vi "acq_loop.vi"(8 "Marker Queue":refnum<queue>, 9 "Log queue":refnum<queue>, 10 "Server queue":refnum<queue>, 11 "Message Queues":T2) -> (0 "error out":errorcluster)   [LabVIEW 2013]
doc: "Message loop for handling messages pertaining to the acquisition of data from the hardware."
uses:
  queues/que_all_message_queues.ctl
  queues/que_message_cluster.ctl
  gui/type_def/device.ctl
  acq_state.ctl
  queues/que_enqueue_message_single.vi
  <vilib>/Utility/error.llb/Error Cluster From Error Code.vi
  <vilib>/ErrorRing/Error Ring.xnode
panel:
  out "eeg_device":T1
  in  "error in (no error)":errorcluster
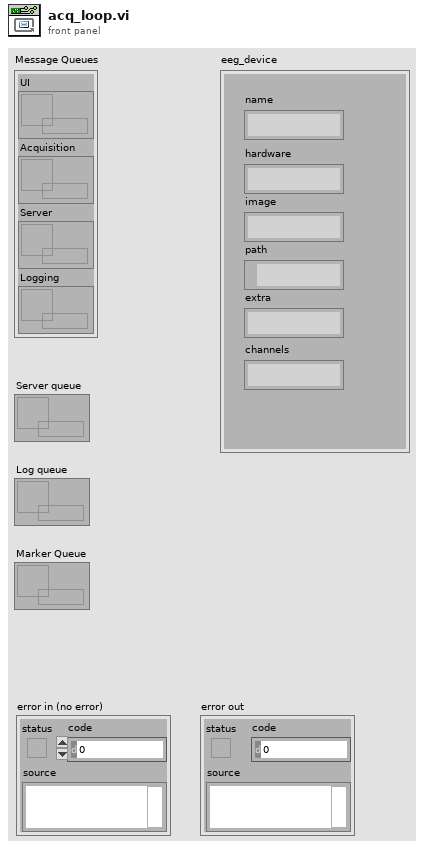
[diagram p1: front panel]
types:
  T1 = typedef "device.ctl" = cluster{"name":string, "hardware":string, "image":string, "path":path, "extra":string, "channels":string}
  T2 = typedef "que_all_message_queues.ctl" = cluster{"UI":refnum<queue>, "Acquisition":refnum<queue>, "Server":refnum<queue>, "Logging":refnum<queue>}
  T3 = typedef "acq_state.ctl" = enum16{"Idle", "Acquiring"}
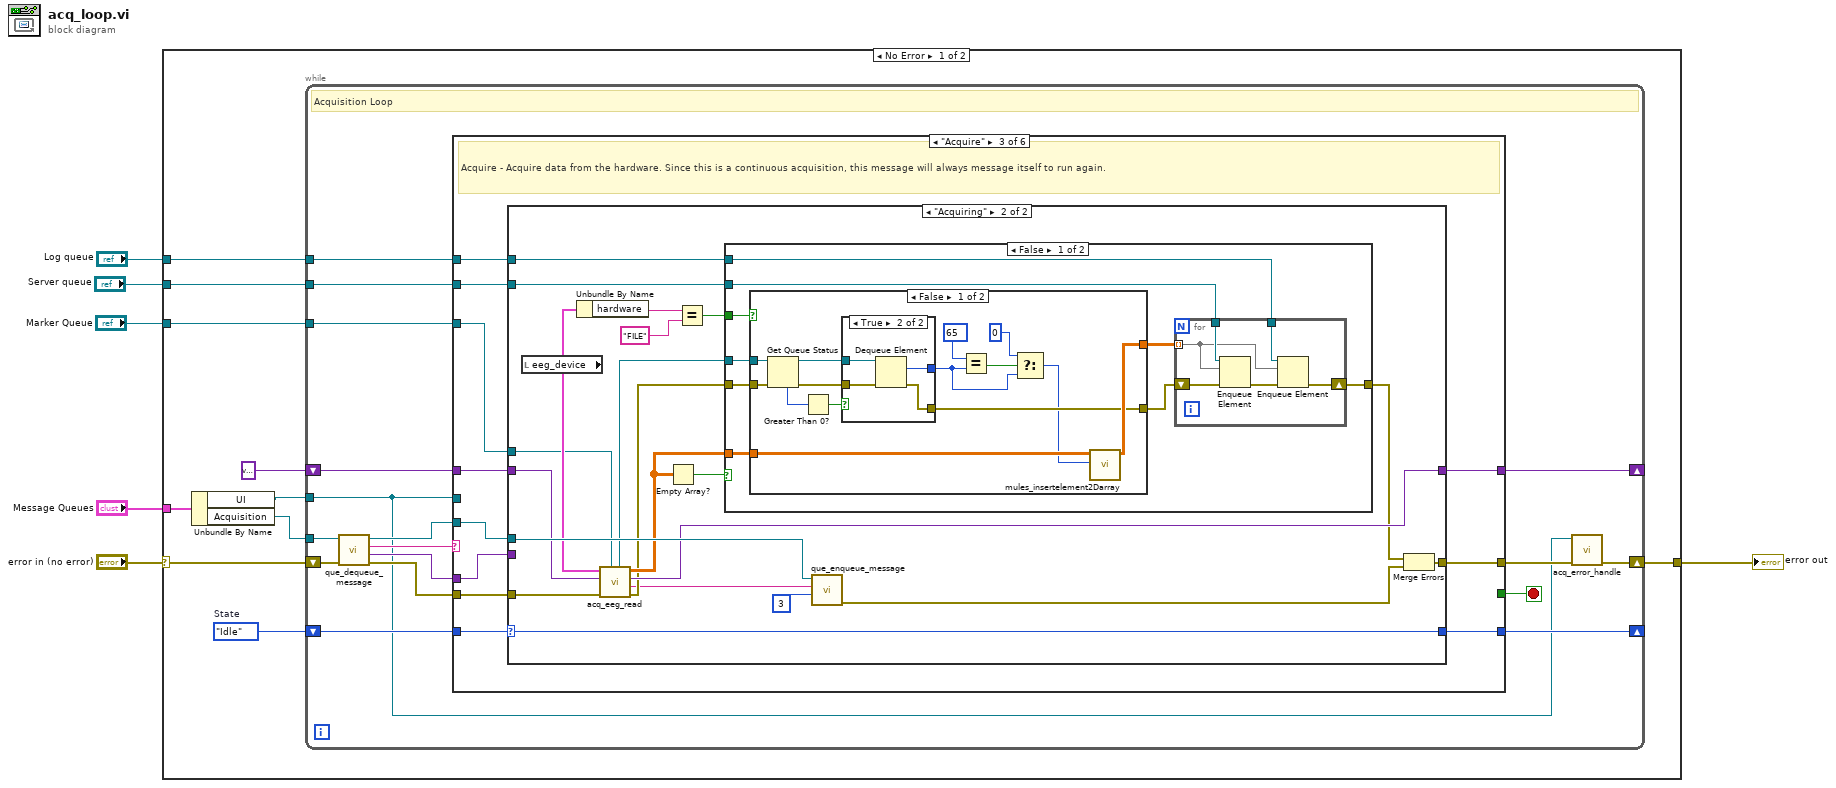
[diagram p0: block diagram]
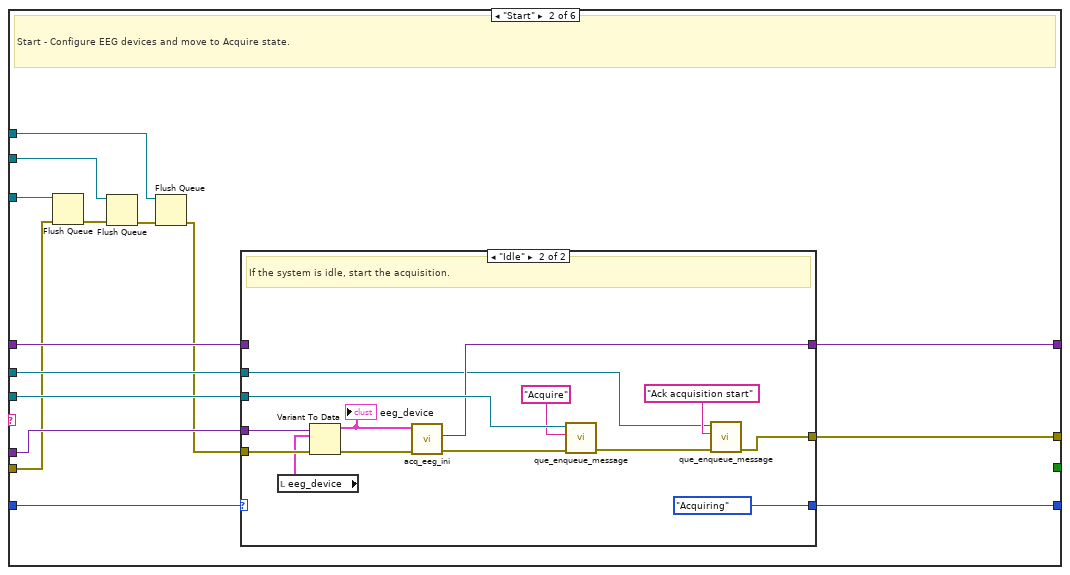
[diagram p3: hidden frame]
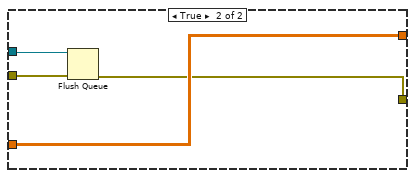
[diagram p7: hidden frame]
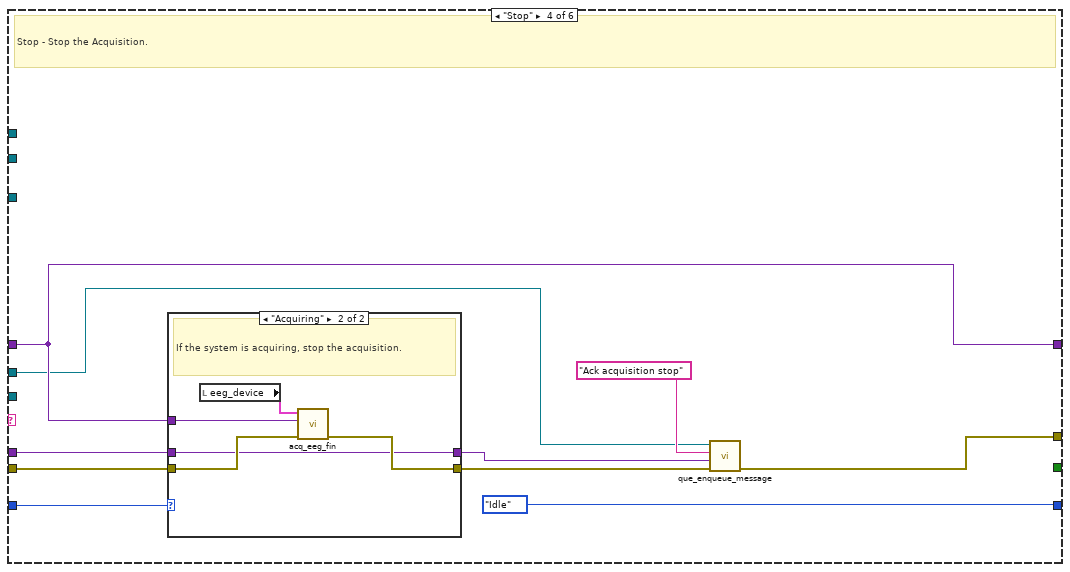
[diagram p9: hidden frame]
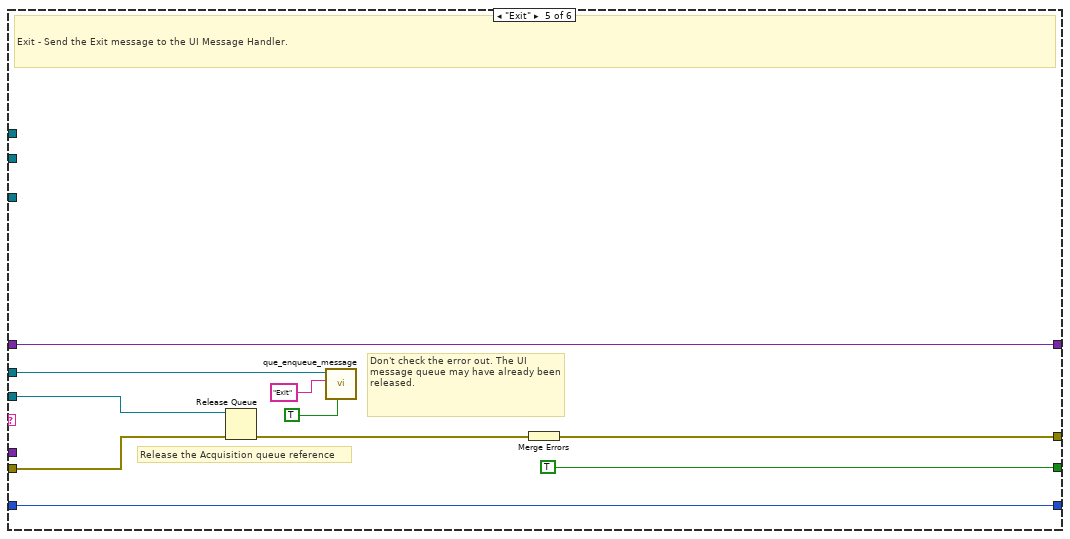
[diagram p11: hidden frame]
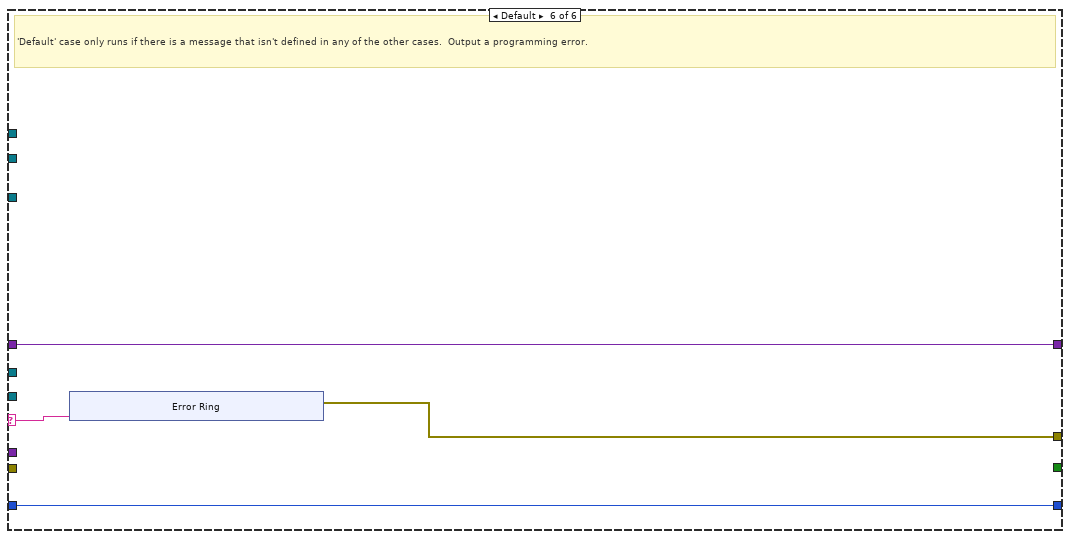
[diagram p12: hidden frame]
diagram:
  n1 = case shown="No Error" "error in (no error)" {
    selector: "error in (no error)" -> [w13 w180]
    tunnel: "Message Queues" -> [w16 _]
    tunnel: [w14 w180] -> w5
    tunnel: "Marker Queue" -> [w9 _]
    tunnel: "Server queue" -> [w8 _]
    tunnel: "Log queue" -> [w7 _]
    frame No Error {
      w11 = acq_state."Idle"  # State
      n2 = Unbundle By Name(w16) -> ("UI"=w12:refnum<queue>, "Acquisition"=w15:refnum<queue>)
      n3 = while {
        tunnel: w15 -> [w28]
        shift-right: [w25] -> w14
        shift-left: w13 -> [w32]
        tunnel: w12 -> [w22]
        shift-right: [w26] -> _
        shift-left: w11 -> [w27]
        shift-right: [w17] -> _
        shift-left: variant ("Variant out") -> [w21]
        tunnel: w9 -> [w20]
        tunnel: w8 -> [w19]
        tunnel: w7 -> [w18]
        stop <- w33 stop-if-true
        # "Acquisition Loop"
        n4 = call "que_dequeue_message.vi"("error in (no error)"=w32, "Message Queue"=w28) -> ("error out"=w31:errorcluster, "Message Data"=w29:variant, "Message"=w30:string, "dup Message Queue"=w23:refnum<queue>)  [unwired: 6 in]
        n5 = case "Message Cases" shown="\"Acquire\"" w30 {
          selector: w30 -> [_ _ _ _ _ w170]
          tunnel: w23 -> [_ w50 w78 _ w161 _]
          tunnel: w31 -> [w34 w39 w77 w151 w165 _]
          tunnel: [w34 w51 w79 w145 w167 w171] -> w24
          tunnel: [_ _ _ _ TRUE _] -> w33
          tunnel: w29 -> [_ w47 w74 w143 _ _]
          tunnel: w22 -> [_ w45 _ w146 w166 _]
          tunnel: w27 -> [w36 w48 w75 w150 w160 w172]
          tunnel: [w36 w49 w76 acq_state."Idle" ("State") w160 w172] -> w26
          tunnel: [w35 w46 w73 w149 w159 w169] -> w17
          tunnel: w21 -> [w35 w44 w72 w149 w159 w169]
          tunnel: w20 -> [_ w42 w71 _ _ _]
          tunnel: w19 -> [_ w43 w70 _ _ _]
          tunnel: w18 -> [_ w41 w69 _ _ _]
          frame "Initialize" {
            # "Initialize  - Initialize is currently a no-op.  The EEG initialization is done with the 'start' message."
          }
          frame "Start" {
            # "Start - Configure EEG devices and move to Acquire state."
            n6 = Flush Queue(queue=w42, error in (no error)=w39) -> (error out=w40:errorcluster)  [unwired: 2 out]
            n7 = Flush Queue(queue=w43, error in (no error)=w40) -> (error out=w38:errorcluster)  [unwired: 2 out]
            n8 = Flush Queue(queue=w41, error in (no error)=w38) -> (error out=w37:errorcluster)  [unwired: 2 out]
            n9 = case shown="\"Idle\"" w48 {
              selector: w48 -> [w53 _]
              tunnel: [w54 w59] -> w51
              tunnel: w37 -> [w54 w64]
              tunnel: w50 -> [_ w68]
              tunnel: [w53 acq_state."Acquiring" ("Acquisition State")] -> w49
              tunnel: w47 -> [_ w65]
              tunnel: [w52 w61] -> w46
              tunnel: w45 -> [_ w58]
              tunnel: w44 -> [w52 _]
              frame "Acquiring" {
                # "The system is already acquiring. Ignore the \"Start\" message."
              }
              frame "Idle" {
                # "If the system is idle, start the acquisition."
                n10 = local read "eeg_device"() -> (w63:T1)
                n11 = Variant To Data(error in=w64, type=w63, Variant=w65) -> (data=w57:T1, error out=w62:errorcluster)
                "eeg_device" <- w57
                n12 = call "acq_eeg_ini.vi"("error in (no error)"=w62, "eeg_device in"=w57) -> ("error out"=w55:errorcluster, "Variant"=w61:variant)  [unwired: 8 in]
                n13 = call-poly "que_enqueue_message.vi"("error in (no error)"=w55, "Message"="Acquire", "Message Queue"=w68) -> ("error out"=w56:errorcluster)  [unwired: 7 in, 1 out]
                n14 = call-poly "que_enqueue_message.vi"("error in (no error)"=w56, "Message"="Ack acquisition start", "Message Queue"=w58) -> ("error out"=w59:errorcluster)  [unwired: 7 in, 1 out]
              }
            }
          }
          frame "Acquire" {
            # "Acquire - Acquire data from the hardware. Since this is a continuous acquisition, this message will always message itself to run again."
            n15 = case shown="\"Acquiring\"" w75 {
              selector: w75 -> [w81 w89]
              tunnel: [w82 w102] -> w79
              tunnel: w78 -> [_ w101]
              tunnel: w77 -> [w82 w96]
              tunnel: [w81 w89] -> w76
              tunnel: w74 -> [_ _]
              tunnel: [w80 w100] -> w73
              tunnel: w72 -> [w80 w99]
              tunnel: w71 -> [_ w88]
              tunnel: w70 -> [_ w95]
              tunnel: w69 -> [_ w85]
              frame "Idle", Default {
                # "Ignore \"Acquire\" messages when the acquisition is idle."
              }
              frame "Acquiring" {
                # "Acquire more data while in the \"Acquiring\" state."
                n16 = local read "eeg_device"() -> (w93:T1)
                n17 = Unbundle By Name(w93) -> ("hardware"=w92:string)
                n18 = call "acq_eeg_read.vi"("Marker Queue"=w88, "error in (no error)"=w96, "variant in"=w99, "eeg_device"=w93) -> ("Next Acq State"=w86:string, "Variant out"=w100:variant, "eeg samples"=w97:dbl[][], "Marker Queue Out"=w87:refnum<queue>)  [unwired: 3 in, 1 out]
                n19 = Empty Array?(array=w97) -> (empty?=w98:bool)
                n20 = Equal?(x=w92, y="FILE" ("Message")) -> (x = y?=w90:bool)
                n21 = case shown="False" w98 {
                  tunnel: w97 -> [w111 _]
                  tunnel: w96 -> [w110 w141]
                  tunnel: w95 -> [w109 _]
                  tunnel: [w107 w141] -> w94
                  tunnel: w90 -> [w106 _]
                  tunnel: w87 -> [w104 _]
                  tunnel: w85 -> [w103 _]
                  frame False {
                    n22 = case shown="False" w106 {
                      tunnel: w111 -> [w131 w140]
                      tunnel: w110 -> [w126 w139]
                      tunnel: [w125 w140] -> w105
                      tunnel: [w124 w138] -> w108
                      tunnel: w104 -> [w123 w137]
                      frame False {
                        n23 = Get Queue Status(queue=w123, error in (no error)=w126) -> (queue out=w128:refnum<queue>, error out=w127:errorcluster, # elements in queue=w130:i32)  [unwired: 1 in, 5 out]
                        n24 = Greater Than 0?(x=w130) -> (x > 0?=w129:bool)
                        n25 = case shown="True" w129 {
                          tunnel: [w132 w136] -> w124
                          tunnel: w128 -> [_ w135]
                          tunnel: [_ w134] -> w120
                          tunnel: w127 -> [w132 w133]
                          frame False {
                          }
                          frame True {
                            n26 = Dequeue Element(queue=w135, error in (no error)=w133) -> (element=w134:u8, error out=w136:errorcluster)  [unwired: 1 in, 2 out]
                          }
                        }
                        n27 = Equal?(x=u8 65 ("y"), y=w120) -> (x = y?=w121:bool)
                        n28 = Select(t=u8 0, s=w121, f=w120) -> (s? t:f=w118:u8)
                        n29 = call "mules_insertelement2Darray.vi"("new element"=w118, "2D array in"=w131) -> ("2D array out"=w125:dbl[][])  [unwired: 9 in]
                      }
                      frame True {
                        n30 = Flush Queue(queue=w137, error in (no error)=w139) -> (error out=w138:errorcluster)  [unwired: 2 out]
                      }
                    }
                    n31 = for {
                      tunnel: w109 -> [w117]
                      tunnel: w105 -> [w113] mode=indexing
                      shift-right: [w112] -> w107
                      shift-left: w108 -> [w116]
                      tunnel: w103 -> [w114]
                      n32 = Enqueue Element(queue=w117, element=w113, error in (no error)=w116) -> (error out=w115:errorcluster)  [unwired: 1 in, 2 out]
                      n33 = Enqueue Element(queue=w114, element=w113, error in (no error)=w115) -> (error out=w112:errorcluster)  [unwired: 1 in, 2 out]
                    }
                  }
                  frame True {
                  }
                }
                n34 = call-poly "que_enqueue_message.vi"("Message Data"=3 ("t"), "Message"=w86, "Message Queue"=w101) -> ("error out"=w83:errorcluster)  [unwired: 7 in, 1 out]
                n35 = Merge Errors(w94, w83) -> (w102:errorcluster)
              }
            }
          }
          frame "Stop" {
            # "Stop - Stop the Acquisition."
            n36 = case shown="\"Acquiring\"" w150 {
              tunnel: w151 -> [w153 w158]
              tunnel: w149 -> [_ w157]
              tunnel: [w153 w155] -> w147
              tunnel: [w152 w154] -> w144
              tunnel: w143 -> [w152 w154]
              frame "Idle", Default {
                # "The system is already idle. Ignore the \"Stop\" message."
              }
              frame "Acquiring" {
                # "If the system is acquiring, stop the acquisition."
                n37 = local read "eeg_device"() -> (w156:T1)
                n38 = call "acq_eeg_fin.vi"("error in (no error)"=w158, "variant in"=w157, "eeg_device"=w156) -> ("error out"=w155:errorcluster)  [unwired: 8 in]
              }
            }
            n39 = call-poly "que_enqueue_message.vi"("error in (no error)"=w147, "Message Data"=w144, "Message"="Ack acquisition stop", "Message Queue"=w146) -> ("error out"=w145:errorcluster)  [unwired: 6 in, 1 out]
          }
          frame "Exit" {
            # "Don't check the error out. The UI message queue may have already been released."
            # "Release the Acquisition queue reference"
            # "Exit - Send the Exit message to the UI Message Handler."
            n40 = Release Queue(queue=w161, error in (no error)=w165) -> (error out=w162:errorcluster)  [unwired: 1 in, 2 out]
            n41 = call-poly "que_enqueue_message.vi"("Priority Message? (F)"=TRUE, "Message"="Exit", "Message Queue"=w166) -> ()  [unwired: 7 in, 2 out]
            n42 = Merge Errors(w162) -> (w167:errorcluster)
          }
          frame Default {
            # "'Default' case only runs if there is a message that isn't defined in any of the other cases.  Output a programming error."
            n43 = xnode "Error Ring"("parameter 0"=w170) -> ("error out"=w171:errorcluster)
          }
        }
        n44 = call "acq_error_handle.vi"("error in (no error)"=w24, "Message Queue"=w22) -> ("dup error in"=w25:errorcluster)  [unwired: 8 in, 1 out]
      }
    }
    frame Error {
    }
  }
  "error out" <- w5
